vi "Publish Result.vi"(8 "error in (no error)":errorcluster, 10 "Results":T1={"Name"="", "Message"="", "Description"="", "Status"=enum."Passed", "Result Type"=enum."Method", "Execution Time"=0.0}, 11 "LUnit Test Suite In":refnum<class "LUnit Test Suite.lvclass">) -> (0 "error out":errorcluster)   [LabVIEW 2020, in "LUnit Test Suite.lvclass"]
uses:
  LUnit Test Suite.lvclass
  Core/Result/Result.ctl
  Core/Result/Status.ctl
  Core/Result/Type.ctl
  LUnit Test Suite.lvclass/LUnit Test Suite.ctl
  Core/Result Observer/Result Observer.lvclass
  Core/Result/Result.lvlib
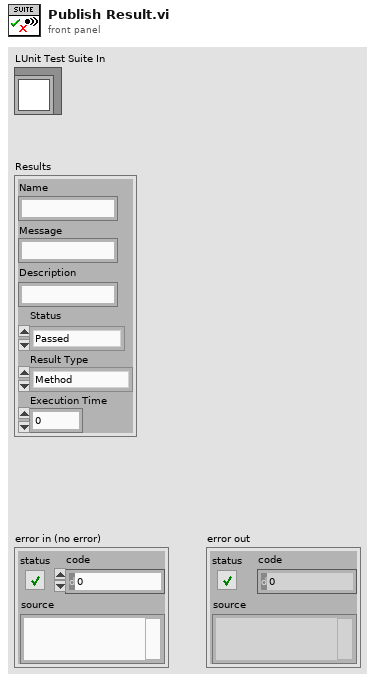
[diagram p1: front panel]
types:
  T1 = typedef "Result.lvlib/Result.ctl" = cluster{"Name":string, "Message":string, "Description":string, "Status":T2, "Result Type":T3, "Execution Time":dbl}
  T2 = typedef "Result.lvlib/Status.ctl" = enum16{"", "Passed", "Failed", "Error", "Skipped", "Setup Error", "Broken", "Teardown Error"}
  T3 = typedef "Result.lvlib/Type.ctl" = enum16{"Method", "Case", "Suite", "Pass", "Fail", "Skip", "Pass if", "Fail if", "Pass if Error", "Fail if Error", "Pass if Equal", "Fail if Equal"}
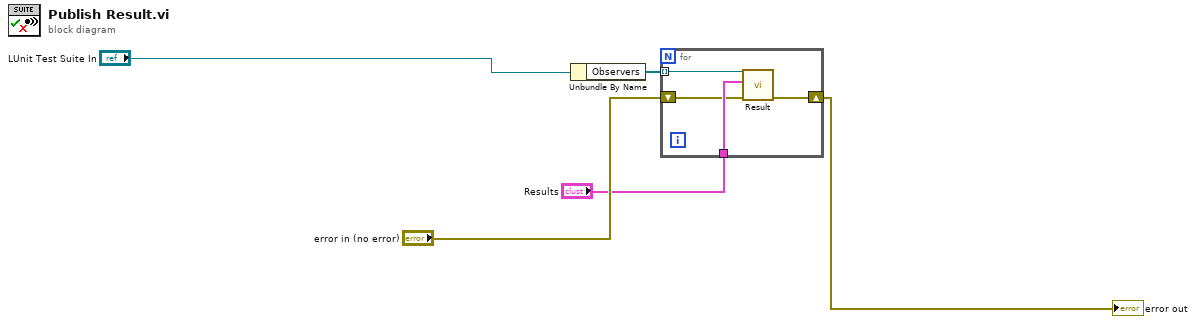
[diagram p0: block diagram]
diagram:
  n1 = Unbundle By Name("LUnit Test Suite In") -> ("Observers"=w5:refnum<class "Result Observer.lvclass">[])
  n2 = for {
    tunnel: "Results" -> [w9]
    shift-right: [w7] -> w3
    shift-left: "error in (no error)" -> [w8]
    tunnel: w5 -> [w6] mode=indexing
    n3 = call-dynamic "Result.vi"("error in (no error)"=w8, "Result"=w9, "Result Observer In"=w6) -> ("error out"=w7:errorcluster)  [unwired: 8 in]
  }
  "error out" <- w3
